vi "JAUS Wrapper.vi"   [LabVIEW 2009]
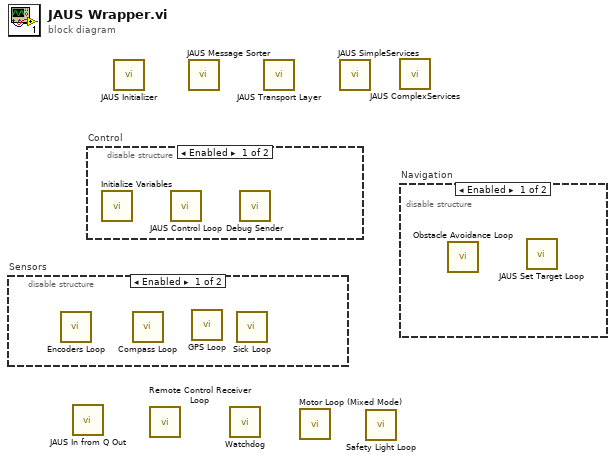
[diagram p0: block diagram]
diagram:
  n1 = disable-structure "Sensors" shown="Enabled" {
    frame #0 {
      n2 = call "Encoders Loop.vi"() -> ()  [unwired: 1 in]
      n3 = call "Compass Loop.vi"() -> ()  [unwired: 1 in]
      n4 = call "GPS Loop.vi"() -> ()  [unwired: 1 in]
      n5 = call "Sick Loop.vi"() -> ()  [unwired: 1 in]
    }
    frame #1 {
    }
  }
  n6 = call "JAUS In from Q Out.vi"() -> ()  [unwired: 1 in]
  n7 = disable-structure "Control" shown="Enabled" {
    frame #0 {
      n8 = call "Initialize Variables.vi"() -> ()  [unwired: 1 in]
      n9 = call "JAUS Control Loop.vi"() -> ()  [unwired: 1 in]
      n10 = call "Debug Sender.vi"() -> ()  [unwired: 1 in]
    }
    frame #1 {
    }
  }
  n11 = call "JAUS Initializer.vi"() -> ()  [unwired: 1 in]
  n12 = call "Remote Control Receiver Loop.vi"() -> ()  [unwired: 1 in]
  n13 = call "JAUS Message Sorter.vi"() -> ()  [unwired: 1 in]
  n14 = call "Watchdog.vi"() -> ()  [unwired: 1 in]
  n15 = call "JAUS Transport Layer.vi"() -> ()  [unwired: 1 in]
  n16 = call "Motor Loop (Mixed Mode).vi"() -> ()  [unwired: 1 in]
  n17 = call "JAUS SimpleServices.vi"() -> ()  [unwired: 1 in]
  n18 = call "Safety Light Loop.vi"() -> ()  [unwired: 1 in]
  n19 = call "JAUS ComplexServices.vi"() -> ()  [unwired: 12 in]
  n20 = disable-structure "Navigation" shown="Enabled" {
    frame #0 {
      n21 = call "Obstacle Avoidance Loop.vi"() -> ()  [unwired: 1 in]
      n22 = call "JAUS Set Target Loop.vi"() -> ()  [unwired: 1 in]
    }
    frame #1 {
    }
  }
